vi "Get All Registered Services.vi"(8 "error in (no error)":errorcluster, 11 "Service in":refnum<class "Service.lvclass">) -> (0 "error out":errorcluster, 2 "Services":string[](array[string]), 3 "Service out":refnum<class "Service.lvclass">)   [LabVIEW 2024, in "Ramses Framework.lvlib" / "Service.lvclass"]
uses:
  Service.lvclass
  Communications/Server/Base Server/Server.lvclass
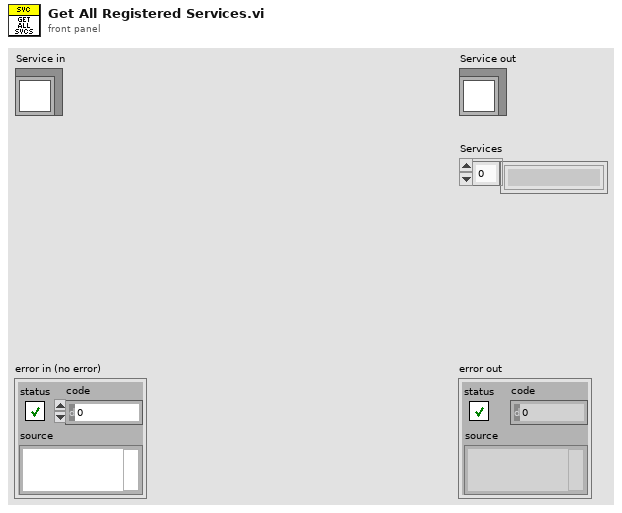
[diagram p1: front panel]
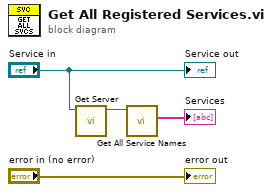
[diagram p0: block diagram]
diagram:
  n1 = call "Get Server.vi"("Service in"="Service in") -> ("Server"=w2:refnum<class "Server.lvclass">)  [unwired: 9 in, 1 out]
  n2 = call-dynamic "Get All Service Names.vi"("Server in"=w2) -> ("Service Names"=→"Services":string[])  [unwired: 8 in, 2 out]
  "error out" <- "error in (no error)"
  "Service out" <- "Service in"
